vi "Exemple_Metrics_Cohen_Kappa_Score.vi"() -> ()   [LabVIEW 2020]
uses:
  Objet/3 - Model selection and evaluation/3.3 - Metrics and scoring/cohen_kappa_score/Cohen_Kappa_Score.vi
panel:
  out "Score":string
  out "error out":errorcluster caption="sortie d'erreur"
  in  "cohen_kappa_score":T1={"labels"=[], "weights"="None", "sample_weight"=[]}
  in  "error in (no error)":errorcluster caption="entrée d'erreur (pas d'erreur)"
  in  "y2":string[][](array[string])=[["0"], ["0"], ["2"], ["2"], ["0"], ["2"]]
  in  "y1":string[][](array[string])=[["2"], ["0"], ["2"], ["2"], ["0"], ["1"]]
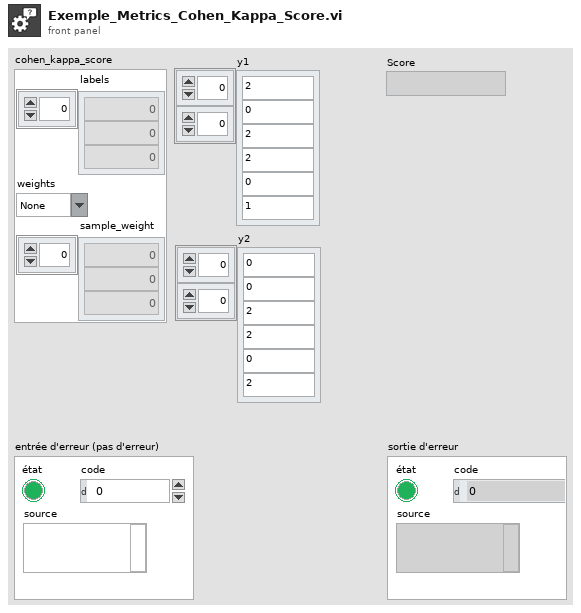
[diagram p1: front panel]
types:
  T1 = cluster{"labels":i32[], "weights":string, "sample_weight":dbl[]}
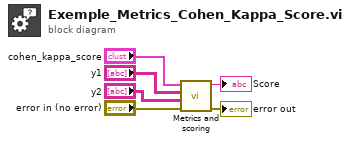
[diagram p0: block diagram]
diagram:
  n1 = call-poly "Metrics and scoring.vi"("error in (no error)"="error in (no error)", "y2"="y2", "y1"="y1", "cohen_kappa_score"="cohen_kappa_score") -> ("error out"=→"error out":errorcluster, "Score"=→"Score":string)  [unwired: 6 in]
